vi "Set Node ID.vi"(10 "Node ID":string, 11 "Node Path":path) -> (3 "File Name Out":string)   [LabVIEW 2020, in "SimpleDependencyInspector.lvlib"]
uses:
  SimpleDependencyInspector.lvlib
  FGV Functions--enum.ctl
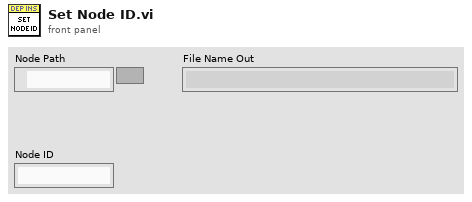
[diagram p1: front panel]
types:
  T1 = typedef "SimpleDependencyInspector.lvlib/FGV Functions--enum.ctl" = enum16{"Initialize", "Get Node ID", "Set Node ID"}
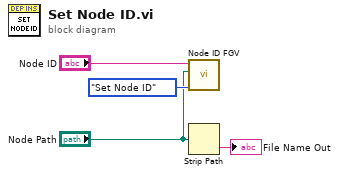
[diagram p0: block diagram]
diagram:
  n1 = call "Node ID FGV.vi"("Initialize"=FGV_Functions--enum."Set Node ID", "Node Path"="Node Path", "Node ID"="Node ID") -> ()  [unwired: 6 in, 3 out]
  n2 = Strip Path(path="Node Path") -> (name=→"File Name Out":string)  [unwired: 1 out]
